vi "OutBit.vi"(7 "CardIndex":i32, 8 "error in (no error)":errorcluster, 10 "BL":bool, 11 "Index":i32) -> (0 "error out":errorcluster)   [LabVIEW 2019]
uses:
  IO_Class/IOCard.lvclass
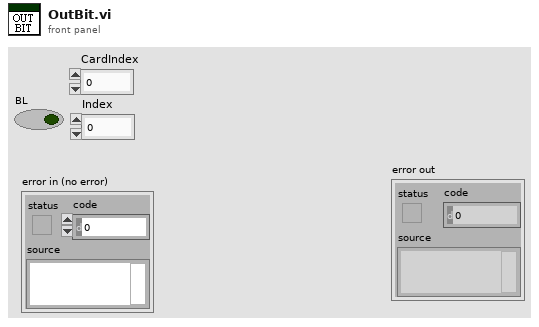
[diagram p1: front panel]
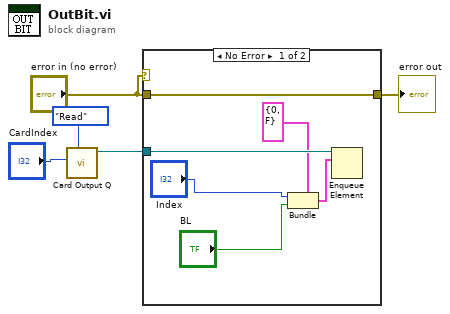
[diagram p0: block diagram]
diagram:
  n1 = call "Card Output Q.vi"("Action"=enum16{"Initial", "Write", "Read", "Release"}."Read", "CardIndex"="CardIndex") -> ("Output Q Out"=w1:refnum<queue>)  [unwired: 8 in, 1 out]
  n2 = case shown="No Error" "error in (no error)" {
    tunnel: "error in (no error)" -> [w10 w12]
    tunnel: [w10 w12] -> w5
    tunnel: w1 -> [w11 _]
    frame No Error {
      n3 = Bundle(cluster=cluster{"Index":i32, "BL":bool} {"Index"=0, "BL"=FALSE} ("element"), "Index"="Index", "BL"="BL") -> (w7:cluster{"Index":i32, "BL":bool})
      n4 = Enqueue Element(queue=w11, element=w7) -> ()  [unwired: 2 in, 3 out]
    }
    frame Error {
    }
  }
  "error out" <- w5
